vi "SetRESTURLandRoot.vi"(8 "error in (no error)":errorcluster, 9 "module":T1, 10 "ByteREST in":refnum<class "RESTBase.lvclass">) -> (0 "error out":errorcluster, 2 "ByteREST out":refnum<class "RESTBase.lvclass">)   [LabVIEW 2019, in "ByteQXWebAPI.lvlib" / "ByteQXAPIBase.lvclass"]
uses:
  ByteQXAPIBase.lvclass
  <vilib>/Bytelabs/ByteREST/ByteRESTClass/ByteRESTBase/RESTBase.lvclass
  module.ctl
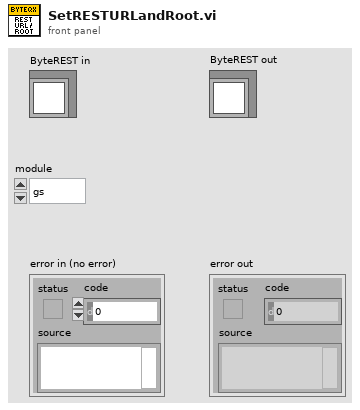
[diagram p1: front panel]
types:
  T1 = typedef "ByteQXWebAPI.lvlib/ByteQXAPIBase.lvclass/module.ctl" = enum16{"gs", "tms", "data"}
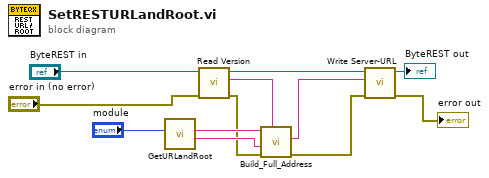
[diagram p0: block diagram]
diagram:
  n1 = call "GetURLandRoot.vi"(10:"module") -> ("API root"=w7:string, "Base URL"=w11:string)  [unwired: 9 in]
  n2 = call-dynamic "Read Version.vi"("error in (no error)"="error in (no error)", "ByteRESTBase in"="ByteREST in") -> ("error out"=w5:errorcluster, "Version"=w9:string, "ByteRESTBase out"=w10:refnum<class "RESTBase.lvclass">)  [unwired: 7 in]
  n3 = call <vilib>:"Build_Full_Address.vi"("Version (no version)"=w9, "error in (no error)"=w5, "API Root"=w7, "Base URL"=w11) -> ("error out"=w4:errorcluster, "Full URL"=w12:string)  [unwired: 6 in]
  n4 = call-dynamic "Write Server-URL.vi"("error in (no error)"=w4, "Server-URL"=w12, "ByteRESTBase in"=w10) -> ("error out"=→"error out":errorcluster, "ByteRESTBase out"=→"ByteREST out":refnum<class "RESTBase.lvclass">)  [unwired: 7 in]
